vi "Write 1Chan NSamp Waveform.vi"(8 "error in (no error)":errorcluster, 10 "data":waveform(dbl), 11 "Analog Output in":refnum<class "Analog output.lvclass">) -> (0 "error out":errorcluster, 3 "Analog Output out":refnum<class "Analog output.lvclass">)   [LabVIEW 2009, in "MicroDAQ.lvlib" / "Analog output.lvclass"]
doc: "Writes waveform to channel."
uses:
  <instrlib>/MicroDAQ/Channel/Analog Output/Analog output.lvclass
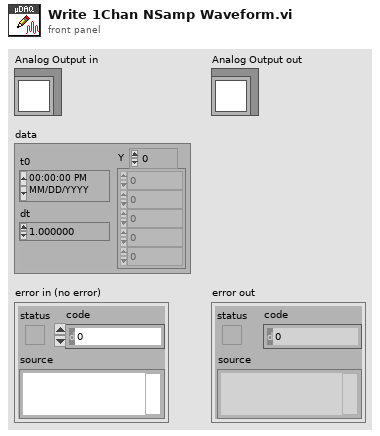
[diagram p1: front panel]
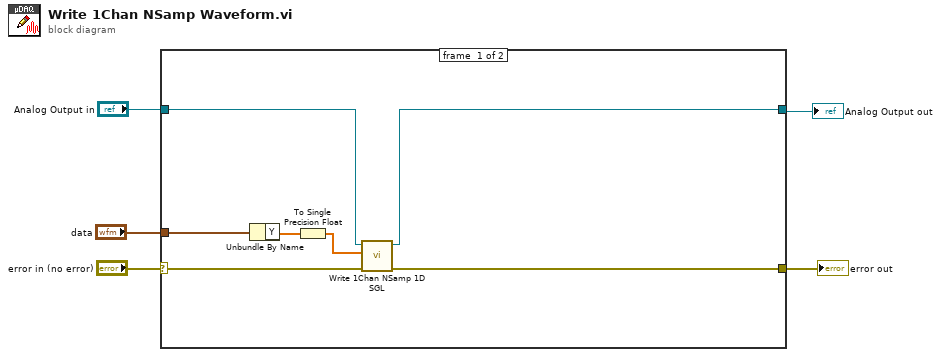
[diagram p0: block diagram]
diagram:
  n1 = case shown="No Error" "error in (no error)" {
    selector: "error in (no error)" -> [w10 w14]
    tunnel: [w9 w14] -> w4
    tunnel: [w8 w13] -> w2
    tunnel: "Analog Output in" -> [w11 w13]
    tunnel: "data" -> [w12 _]
    frame #0 {
      n2 = Unbundle By Name(w12) -> ("Y"=w7:dbl[])
      n3 = To Single Precision Float(number=w7) -> (single precision float=w6:sgl[])
      n4 = call <instrlib>:"Write 1Chan NSamp 1D SGL.vi"("error in (no error)"=w10, "data"=w6, "Analog Output in"=w11) -> ("error out"=w9:errorcluster, "Analog Output out"=w8:refnum<class "Analog output.lvclass">)  [unwired: 7 in]
    }
    frame #1 {
    }
  }
  "error out" <- w4
  "Analog Output out" <- w2
